vi "Latest Value Channel Page.vi"(8 "error in (no error)":errorcluster, 11 "Node Ptr":T1 format="%.0x") -> (0 "error out":errorcluster)   [LabVIEW 2015, in "Waveform-Processing-Custom-Device System Explorer.lvlib"]
uses:
  Waveform-Processing-Custom-Device System Explorer.lvlib
  <vilib>/NI Veristand/Custom Device API/Custom Device Item Ref.ctl
  <vilib>/NI VeriStand/Custom Device API/Custom Device API.lvlib
panel:
  in  "SHDocVw.IWebBrowser":refnum<k7>(container)
  in  "Specific Header":cluster{"Section Name":string}={"Section Name"="Specific Page Settings"}
  in  "General Header":cluster{"Section Name":string}={"Section Name"="General Page Settings"}
  in  "Description":string
  in  "Name":string
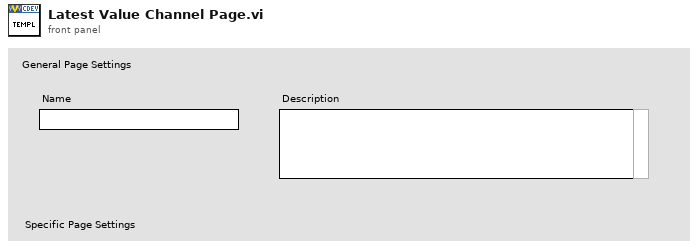
[diagram p1: front panel]
types:
  T1 = typedef "Custom Device API.lvlib/Custom Device Item Ref.ctl" = u64
  T2 = typedef "Custom Device API.lvlib/Custom Device Item Info.ctl" = cluster{"Name":string, "Is Channel":bool, "GUID":string, "Is Waveform":bool}
  T3 = typedef "Custom Device API.lvlib/Custom Device Commands.ctl" = enum16{"Default", "Item renamed", "Shutdown", "Dynamic button pressed"}
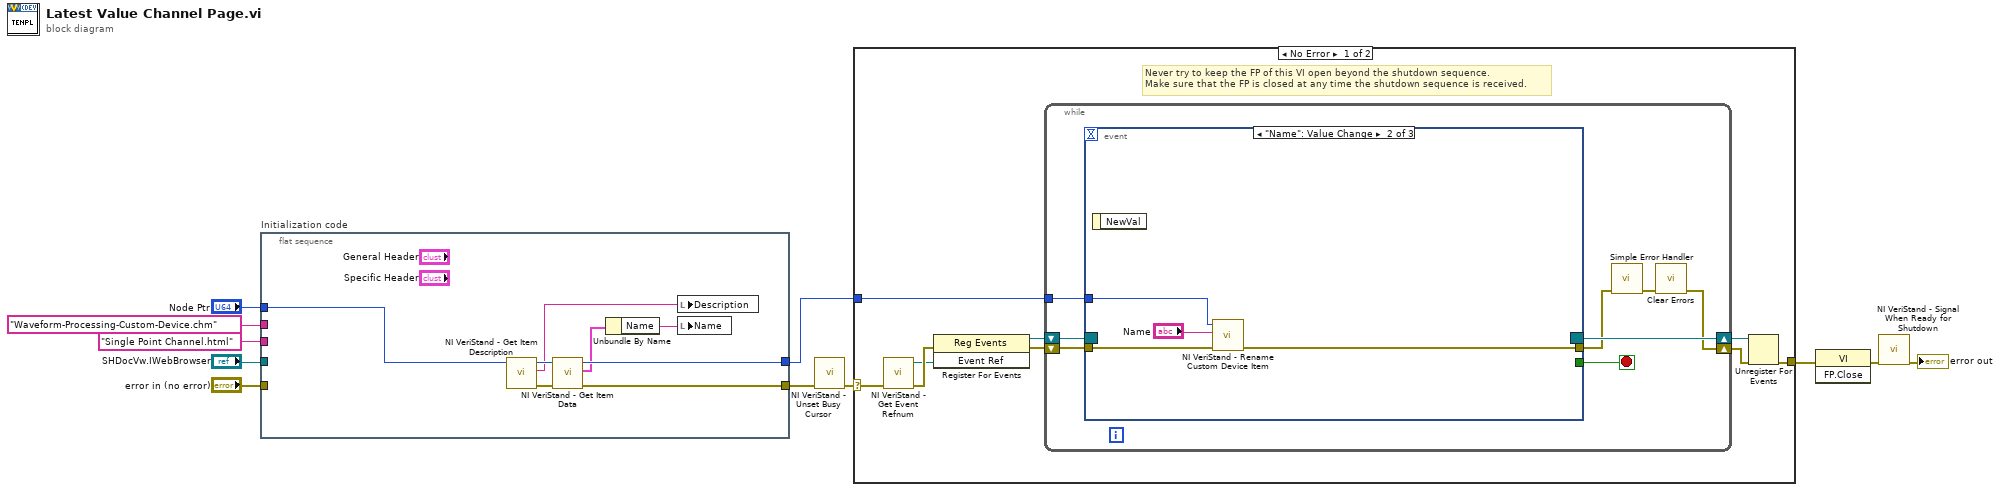
[diagram p0: block diagram]
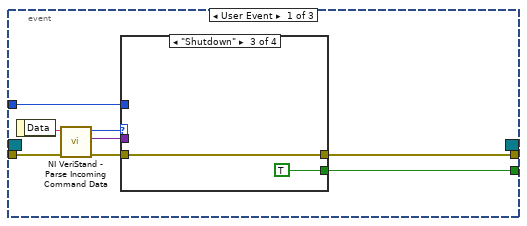
[diagram p2: hidden frame]
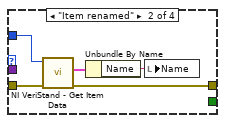
[diagram p4: hidden frame]
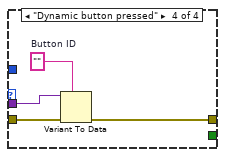
[diagram p5: hidden frame]
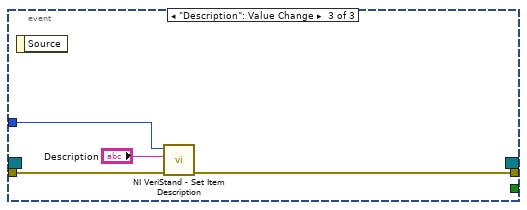
[diagram p6: hidden frame]
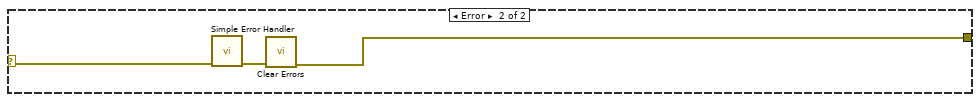
[diagram p7: hidden frame]
diagram:
  n1 = flat-sequence "Initialization code" {
    tunnel: "error in (no error)" -> [_]
    tunnel: "Node Ptr" -> [w14]
    tunnel: [w15] -> w7
    tunnel: [w19] -> w4
    tunnel: "SHDocVw.IWebBrowser" -> [_]
    tunnel: "Single Point Channel.html" ("CD_CHM_Section") -> [_]
    tunnel: "Waveform-Processing-Custom-Device.chm" ("CD_CHM_FileName") -> [_]
    frame #0 {
      n2 = call <vilib>:"NI VeriStand - Get Item Description.vi"("Item Ref in"=w14) -> ("error out"=w17:errorcluster, "Description"=w12:string, "Item Ref out"=w18:T1)  [unwired: 1 in, 7 out]
      n3 = call <vilib>:"NI VeriStand - Get Item Data.vi"("error in (no error)"=w17, "Item Ref in"=w18) -> ("error out"=w15:errorcluster, "Item Info"=w16:T2, "Item Ref out"=w19:T1)  [unwired: 7 out]
      n4 = Unbundle By Name(w16) -> ("Name"=w13:string)
      n5 = local write "Description"(w12) -> ()
      n6 = local write "Name"(w13) -> ()
    }
  }
  n7 = call <vilib>:"NI VeriStand - Unset Busy Cursor.vi"("error in (no error)"=w7) -> ("error out"=w6:errorcluster)  [unwired: 10 out]
  n8 = case shown="No Error" w6 {
    selector: w6 -> [w20 w67]
    tunnel: [w25 w65] -> w11
    tunnel: w4 -> [w21 _]
    frame No Error {
      # "Never try to keep the FP of this VI open beyond the shutdown sequence.\nMake sure that the FP is closed at any time the shutdown sequence is received."
      n9 = call <vilib>:"NI VeriStand - Get Event Refnum.vi"("error in (no error)"=w20) -> ("error out"=w28:errorcluster, "Event Ref"=w24:refnum<user-event>)  [unwired: 9 out]
      n10 = register-events(error in=w28, w24) -> (reference out=w22:refnum<event-registration>, error out=w23:errorcluster)  [unwired: 1 in]
      n11 = while {
        tunnel: w21 -> [w32]
        shift-right: [w29] -> w26
        shift-left: w23 -> [w35]
        shift-right: [w36] -> w27
        shift-left: w22 -> [w34]
        stop <- w33 stop-if-true
        n12 = event shown="[1] \"Name\": Value Change" {
          selector: w34 -> [_ _ _]
          dyn-events: [_ _ _] -> w36
          timeout: _ -> [_ _ _]
          tunnel: w35 -> [w44 w60 w63]
          tunnel: [w40 _ _] -> w33
          tunnel: [w39 w59 w62] -> w31
          tunnel: w32 -> [w38 w58 w64]
          event User Event {
            n13 = event-data() -> ("Data"=w43:string)  [unwired: 1 out]
            n14 = call <vilib>:"NI VeriStand - Parse Incoming Command Data.vi"("error in (no error)"=w44, "Incoming data"=w43) -> ("error out"=w42:errorcluster, "Outgoing data"=w37:variant, "Action"=w41:T3)  [unwired: 7 out]
            n15 = case shown="\"Shutdown\"" w41 {
              tunnel: w42 -> [w45 w50 w51 w56]
              tunnel: [_ _ TRUE _] -> w40
              tunnel: [w45 w47 w51 w53] -> w39
              tunnel: w38 -> [_ w49 _ _]
              tunnel: w37 -> [_ _ _ w55]
              frame "Default", Default {
              }
              frame "Item renamed" {
                n16 = call <vilib>:"NI VeriStand - Get Item Data.vi"("error in (no error)"=w50, "Item Ref in"=w49) -> ("error out"=w47:errorcluster, "Item Info"=w48:T2)  [unwired: 8 out]
                n17 = Unbundle By Name(w48) -> ("Name"=w46:string)
                n18 = local write "Name"(w46) -> ()
              }
              frame "Shutdown" {
              }
              frame "Dynamic button pressed" {
                w54 = ""  # Button ID
                n19 = Variant To Data(error in=w56, type=w54, Variant=w55) -> (error out=w53:errorcluster)  [unwired: 1 out]
              }
            }
          }
          event "Name": Value Change {
            n20 = event-data() -> ()  [unwired: 2 out]
            n21 = call <vilib>:"NI VeriStand - Rename Custom Device Item.vi"("error in (no error)"=w60, "New Name"="Name", "Item Ref in"=w58) -> ("error out"=w59:errorcluster)  [unwired: 1 in, 7 out]
          }
          event "Description": Value Change {
            n22 = event-data() -> ()  [unwired: 2 out]
            n23 = call <vilib>:"NI VeriStand - Set Item Description.vi"("error in (no error)"=w63, "Description"="Description", "Item Ref in"=w64) -> ("error out"=w62:errorcluster)  [unwired: 8 out]
          }
        }
        n24 = call <vilib>:"Simple Error Handler.vi"("error in (no error)"=w31) -> ("error out"=w30:errorcluster)  [unwired: 1 in, 7 out]
        n25 = call <vilib>:"Clear Errors.vi"("error in (no error)"=w30) -> ("error out"=w29:errorcluster)  [unwired: 1 in, 5 out]
      }
      n26 = Unregister For Events(event registration refnum=w27, error in=w26) -> (error out=w25:errorcluster)
    }
    frame Error {
      n27 = call <vilib>:"Simple Error Handler.vi"("error in (no error)"=w67) -> ("error out"=w66:errorcluster)  [unwired: 1 in, 7 out]
      n28 = call <vilib>:"Clear Errors.vi"("error in (no error)"=w66) -> ("error out"=w65:errorcluster)  [unwired: 1 in, 5 out]
    }
  }
  n29 = invoke class="VI" method="FP.Close"(error in=w11) -> (error out=w10:errorcluster)  [unwired: 2 in, 2 out]
  n30 = call <vilib>:"NI VeriStand - Signal When Ready for Shutdown.vi"("error in (no error)"=w10) -> ("error out"=→"error out":errorcluster)  [unwired: 10 out]
